vi "Handle Notification.vi"(8 "error in (no error)":errorcluster, 9 "Payload":string, 10 "Notification Type":string, 11 "Test Sequencer in":refnum<class "Sequencer with Output Values.lvclass">) -> (0 "error out":errorcluster, 3 "Test Sequencer out":refnum<class "Sequencer with Output Values.lvclass">)   [LabVIEW 2020, in "Sequencer with Output Values.lvlib" / "Sequencer with Output Values.lvclass"]
uses:
  Sequencer with Output Values.lvclass
  Sequencer with Output Values.lvclass/Sequencer with Output Values.ctl
  Global Strings.vi
  <vilib>/FlexLogger/SDK/PluginSDK.lvlibp
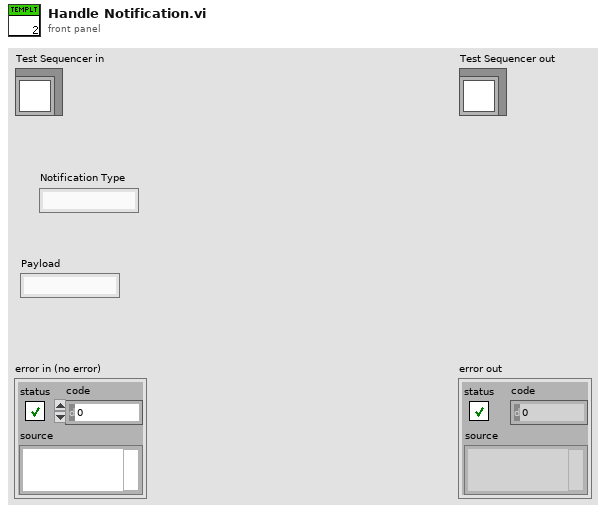
[diagram p1: front panel]
types:
  T1 = typedef "Sequencer with Output Values.lvlib/Sequencer with Output Values.lvclass/Params.ctl" = cluster{"Step Values":T2[], "Only Execute When Test Running":bool, "Reset Sequence When Test Starts":bool, "Current Sequence ID":u32, "Total Iterations":u32, "Current Step Start Timestamp":dbl, "Number of Sequence Steps":i32, "Num of Analog Channels":i32, "Num of Digital Channels":i32, "Delay Before Starting Sequence":dbl, "Show UI":bool, "Time Remaining":dbl, "Test Running":bool, "Pause Timestamp":dbl}
  T2 = typedef "Sequencer with Output Values.lvlib/Sequencer with Output Values.lvclass/Step Settings.ctl" = cluster{"Duration":dbl, "Mode":string, "Delay Between Values":dbl, "Analog Values":string[], "Digital Values":string[]}
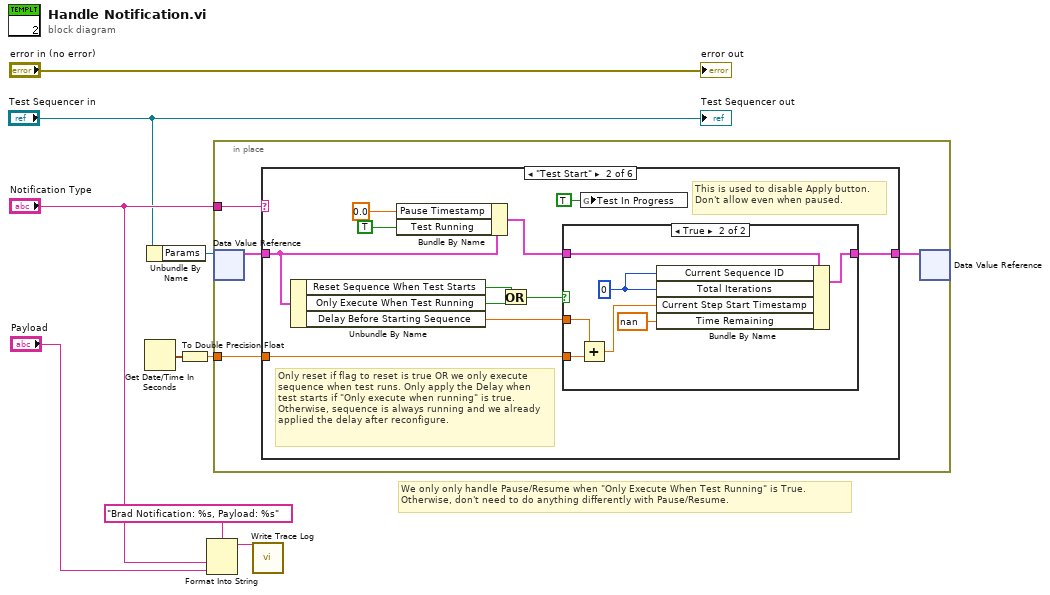
[diagram p0: block diagram]
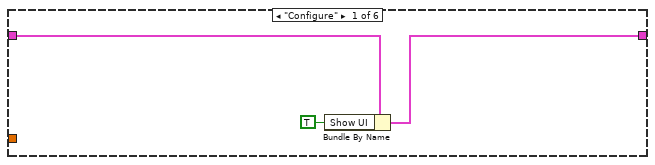
[diagram p2: hidden frame]
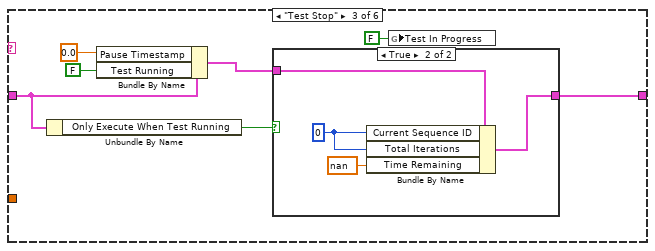
[diagram p4: hidden frame]
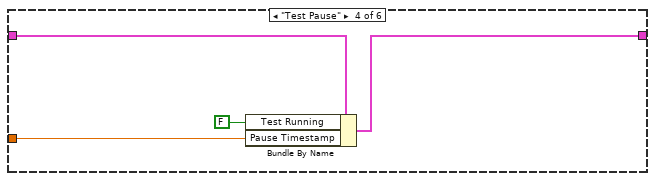
[diagram p6: hidden frame]
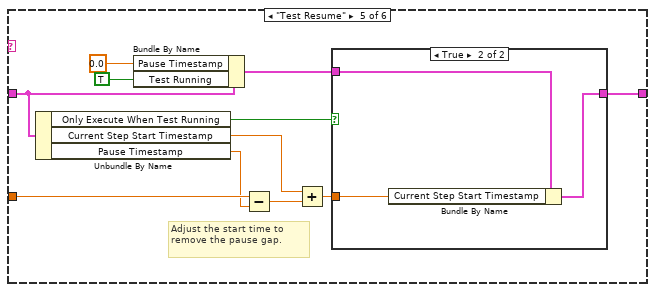
[diagram p7: hidden frame]
diagram:
  # "We only only handle Pause/Resume when \"Only Execute When Test Running\" is True.\nOtherwise, don't need to do anything differently with Pause/Resume."
  n1 = Get Date/Time In Seconds() -> (seconds since 1Jan1904=w2:timestamp)
  n2 = Unbundle By Name("Test Sequencer in") -> ("Params"=w3:refnum<data-value>)
  n3 = To Double Precision Float(number=w2) -> (double precision float=w1:dbl)
  n4 = Format Into String(format string="Brad Notification: %s, Payload: %s", "Notification Type", "Payload") -> (resulting string=w8:string)  [unwired: 2 in, 1 out]
  n5 = in-place {
    in-place-border: "Notification Type" -> [w13]
    in-place-border: w1 -> [w10]
    n6 = in-place-dvr #1(w3) -> (w12:T1)  [unwired: 1 out]
    n7 = case shown="\"Test Start\"" w13 {
      tunnel: w12 -> [w15 w23 w41 w50 w61 w67]
      tunnel: [w14 w22 w38 w49 w55 w67] -> w11
      tunnel: w10 -> [_ w21 _ w48 w60 _]
      frame "Configure" {
        n8 = Bundle By Name(cluster=w15, "Show UI"=TRUE) -> (w14:T1)
      }
      frame "Test Start" {
        # "This is used to disable Apply button. Don't allow even when paused."
        # "Only reset if flag to reset is true OR we only execute sequence when test runs. Only apply the Delay when test starts if \"Only execute when running\" is true. Otherwise, sequence is always running and we already applied the delay after reconfigure."
        n9 = Unbundle By Name(w23) -> ("Reset Sequence When Test Starts"=w25:bool, "Only Execute When Test Running"=w18:bool, "Delay Before Starting Sequence"=w17:dbl)
        n10 = Bundle By Name(cluster=w23, "Pause Timestamp"=0.0, "Test Running"=TRUE) -> (w26:T1)
        n11 = Or(x=w25, y=w18) -> (x .or. y?=w24:bool)
        n12 = case shown="True" w24 {
          tunnel: [w28 w35] -> w22
          tunnel: w26 -> [w28 w33]
          tunnel: w21 -> [_ w32]
          tunnel: w17 -> [_ w31]
          frame False {
          }
          frame True {
            w34 = u32 0 ("Total Iterations")
            n13 = Add(x=w31, y=w32) -> (x+y=w30:dbl)
            n14 = Bundle By Name(cluster=w33, "Current Sequence ID"=w34, "Total Iterations"=w34, "Current Step Start Timestamp"=w30, "Time Remaining"=nan) -> (w35:T1)
          }
        }
        n15 = global write "Global Strings.vi" "Test In Progress"(TRUE ("Test In Progress")) -> ()
      }
      frame "Test Stop" {
        n16 = Unbundle By Name(w41) -> ("Only Execute When Test Running"=w40:bool)
        n17 = Bundle By Name(cluster=w41, "Pause Timestamp"=0.0, "Test Running"=FALSE) -> (w39:T1)
        n18 = case shown="True" w40 {
          tunnel: w39 -> [w43 w47]
          tunnel: [w43 w45] -> w38
          frame False {
          }
          frame True {
            w46 = u32 0 ("Current Sequence ID")
            n19 = Bundle By Name(cluster=w47, "Current Sequence ID"=w46, "Total Iterations"=w46, "Time Remaining"=nan) -> (w45:T1)
          }
        }
        n20 = global write "Global Strings.vi" "Test In Progress"(FALSE ("Test In Progress")) -> ()
      }
      frame "Test Pause" {
        n21 = Bundle By Name(cluster=w50, "Test Running"=FALSE, "Pause Timestamp"=w48) -> (w49:T1)
      }
      frame "Test Resume" {
        # "Adjust the start time to remove the pause gap."
        n22 = Unbundle By Name(w61) -> ("Only Execute When Test Running"=w53:bool, "Current Step Start Timestamp"=w58:dbl, "Pause Timestamp"=w59:dbl)
        n23 = Bundle By Name(cluster=w61, "Pause Timestamp"=0.0, "Test Running"=TRUE) -> (w57:T1)
        n24 = Subtract(x=w60, y=w59) -> (x-y=w54:dbl)
        n25 = Add(x=w58, y=w54) -> (x+y=w56:dbl)
        n26 = case shown="True" w53 {
          tunnel: w57 -> [w63 w66]
          tunnel: w56 -> [_ w65]
          tunnel: [w63 w64] -> w55
          frame False {
          }
          frame True {
            n27 = Bundle By Name(cluster=w66, "Current Step Start Timestamp"=w65) -> (w64:T1)
          }
        }
      }
      frame Default {
      }
    }
    n28 = in-place-dvr #1(w11) -> ()  [unwired: 2 out]
  }
  n29 = call <vilib>:"Write Trace Log.vi"("Message"=w8) -> ()  [unwired: 10 in, 1 out]
  "error out" <- "error in (no error)"
  "Test Sequencer out" <- "Test Sequencer in"
